vi "Log_df.vi"(8 "error in":errorcluster, 9 "seconds since 1Jan1904":timestamp, 10 "df":sgl, 11 "df_Refs":T1 {"Filter_Group_ref" format="%.0x"; "TimeStamp_dset" format="%.0x"; "Filter_dset" format="%.0x"}) -> (0 "error out":errorcluster)   [LabVIEW 2018]
uses:
  HDF5_Filter_refs.ctl
  <vilib>/addons/h5labview2/base/hid_t.ctl
  lib_path_mod_20200519.vi
  <vilib>/addons/h5labview2/base/H5Equery.vi
  <vilib>/addons/h5labview2/dataset/H5Dwrite.llb/H5Dwrite.xnode
  <vilib>/addons/h5labview2/dataset/H5D.lvlib
  <vilib>/addons/h5labview2/space/H5S.lvlib
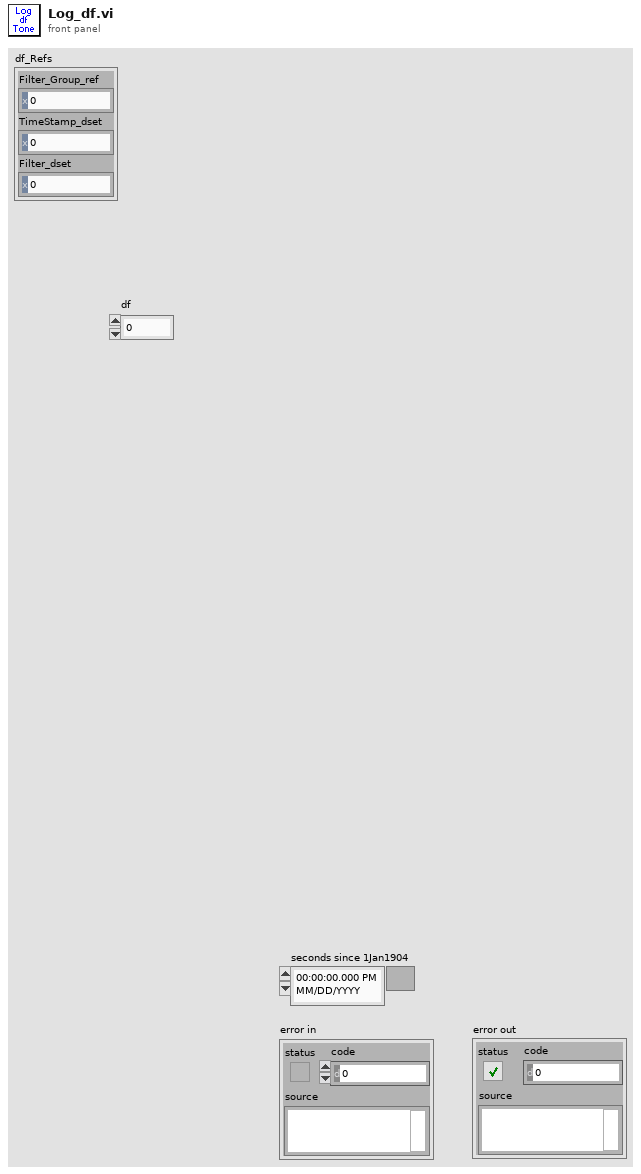
[diagram p1: front panel]
types:
  T1 = typedef "HDF5_Filter_refs.ctl" = cluster{"Filter_Group_ref":T2, "TimeStamp_dset":T2, "Filter_dset":T2}
  T2 = typedef "hid_t.ctl" = i32
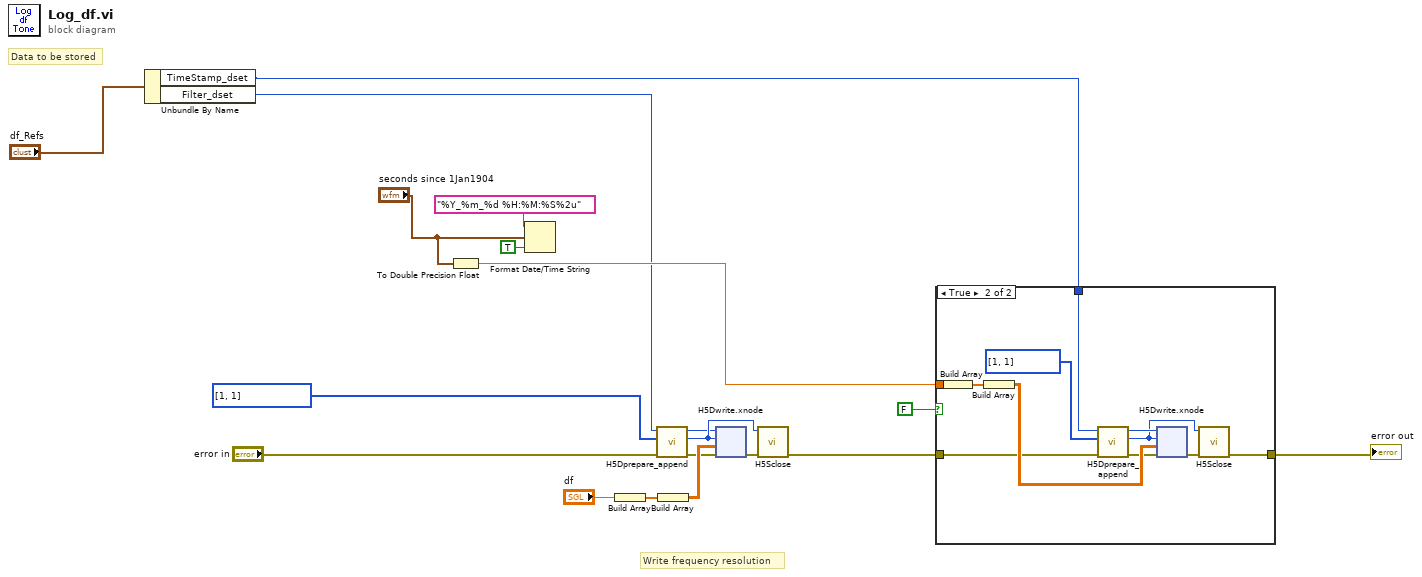
[diagram p0: block diagram]
diagram:
  # "Write frequency resolution"
  # "Data to be stored"
  n1 = Unbundle By Name("df_Refs") -> ("TimeStamp_dset"=w16:T2, "Filter_dset"=w17:T2)
  n2 = To Double Precision Float(number="seconds since 1Jan1904") -> (double precision float=w19:dbl)
  n3 = Format Date/Time String(time format string (%c)="%Y_%m_%d %H:%M:%S%2u", seconds (now)="seconds since 1Jan1904", UTC format=TRUE) -> ()  [unwired: 1 out]
  n4 = Build Array("df") -> (w1:sgl[])
  n5 = call <vilib>:"H5Dprepare_append.vi"("error in (no error)"="error in", "append dims"=u64[] [1, 1], "dset in"=w17) -> ("error out"=w12:errorcluster, "space out"=w14:T2, "dset out"=w13:T2)  [unwired: 5 in, 1 out]
  n6 = Build Array(w1) -> (w18:sgl[][])
  n7 = xnode "H5Dwrite.xnode"("error in (no error)"=w12, "data"=w18, "file space"=w14, "ref in"=w13) -> ("error out"=w11:errorcluster)  [unwired: 3 in, 2 out]
  n8 = call <vilib>:"H5Sclose.vi"("error in (no error)"=w11, "space in"=w14) -> ("error out"=w15:errorcluster)  [unwired: 9 in]
  n9 = case shown="True" FALSE ("LogTime?") {
    tunnel: w19 -> [_ w31]
    tunnel: w16 -> [_ w29]
    tunnel: w15 -> [w20 w28]
    tunnel: [w20 w21] -> w6
    frame False {
      # "Probably don't need to log the time column.\nI'm going to wait until Nick sees and approves\nbefore removing this.\nLuke\n12-19-2018"
    }
    frame True {
      n10 = Build Array(w31) -> (w25:dbl[])
      n11 = Build Array(w25) -> (w30:dbl[][])
      n12 = call <vilib>:"H5Dprepare_append.vi"("error in (no error)"=w28, "append dims"=u64[] [1, 1], "dset in"=w29) -> ("error out"=w26:errorcluster, "space out"=w23:T2, "dset out"=w24:T2)  [unwired: 5 in, 1 out]
      n13 = xnode "H5Dwrite.xnode"("error in (no error)"=w26, "data"=w30, "file space"=w23, "ref in"=w24) -> ("error out"=w27:errorcluster)  [unwired: 3 in, 2 out]
      n14 = call <vilib>:"H5Sclose.vi"("error in (no error)"=w27, "space in"=w23) -> ("error out"=w21:errorcluster)  [unwired: 9 in]
    }
  }
  "error out" <- w6
